vi "CloseExporterConfigurationPageRefs.vi"(8 "error in (no error)":errorcluster, 11 "UIManager in":refnum<class "UIManager.lvclass">) -> (0 "error out":errorcluster, 3 "UIManager out":refnum<class "UIManager.lvclass">)   [LabVIEW 2020, in "UserInterface.lvlib" / "UIManager.lvclass"]
uses:
  UIManager.lvclass
  UIManager.lvclass/UIManager.ctl
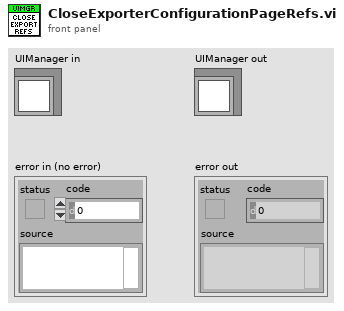
[diagram p1: front panel]
types:
  T1 = typedef "UserInterface.lvlib/UIManager.lvclass/subReferenceData.ctl" = cluster{"VI Ref":refnum<vi>, "Stop":refnum<user-event>, "Parameters":refnum<user-event>}
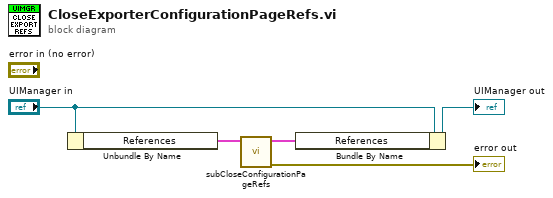
[diagram p0: block diagram]
diagram:
  n1 = Unbundle By Name("UIManager in") -> ("References"=w5:T1)
  n2 = call "subCloseConfigurationPageRefs.vi"("References"=w5) -> ("error out"=→"error out":errorcluster, "Rule parser info.References"=w2:T1)  [unwired: 9 in]
  n3 = Bundle By Name(cluster="UIManager in", "References"=w2) -> (→"UIManager out":refnum<class "UIManager.lvclass">)
